vi "Split and Enqueue.vi"(8 "error in (no error)":errorcluster, 10 "Input String":string, 11 "queue in":refnum<queue>) -> (0 "error out":errorcluster, 3 "queue out":refnum<queue>)   [LabVIEW 2013]
doc: "This sub-VI splits a multi-line input string into an array of single-line strings, and enqueues each element\nof the array into a string queue."
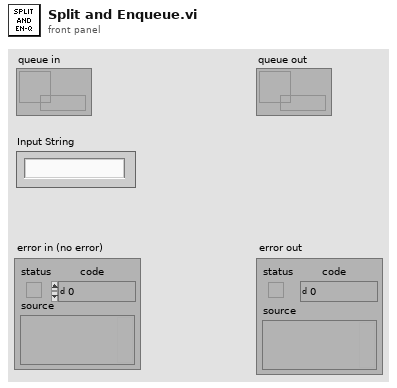
[diagram p1: front panel]
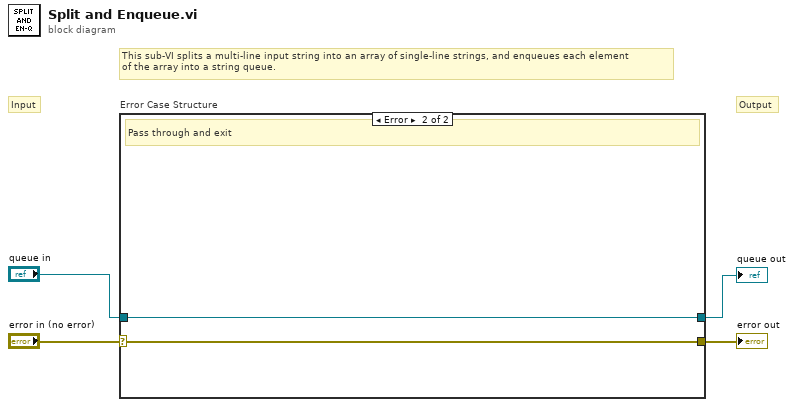
[diagram p0: block diagram]
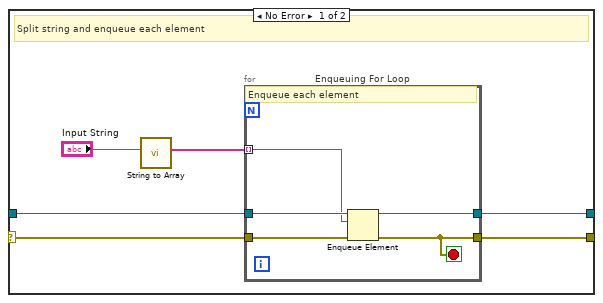
[diagram p2: hidden frame]
diagram:
  # "Output"
  # "Input"
  # "This sub-VI splits a multi-line input string into an array of single-line strings, and enqueues each element\nof the array into a string queue."
  n1 = case "Error Case Structure" shown="Error" "error in (no error)" {
    selector: "error in (no error)" -> [w9 w17]
    tunnel: [w8 w17] -> w3
    tunnel: "queue in" -> [w7 w16]
    tunnel: [w6 w16] -> w1
    frame No Error {
      # "Split string and enqueue each element"
      n2 = call "String to Array.vi"("Input String"="Input String") -> ("String Array"=w5:string[])  [unwired: 10 in]
      n3 = for "Enqueuing For Loop" {
        tunnel: w9 -> [w15]
        tunnel: [w14] -> w8
        tunnel: w7 -> [w13]
        tunnel: [w12] -> w6
        tunnel: w5 -> [w11] mode=indexing
        stop <- w14 stop-if-true
        # "Enqueue each element"
        n4 = Enqueue Element(queue=w13, element=w11, error in (no error)=w15) -> (queue out=w12:refnum<queue>, error out=w14:errorcluster)  [unwired: 1 in, 1 out]
      }
    }
    frame Error {
      # "Pass through and exit"
    }
  }
  "error out" <- w3
  "queue out" <- w1
